vi "random_average_activity_11.vi"() -> ()   [LabVIEW 2025]
panel:
  in  "Enable":bool
  out "RandomSignal":dbl(graph)
  # "off"
  # "on"
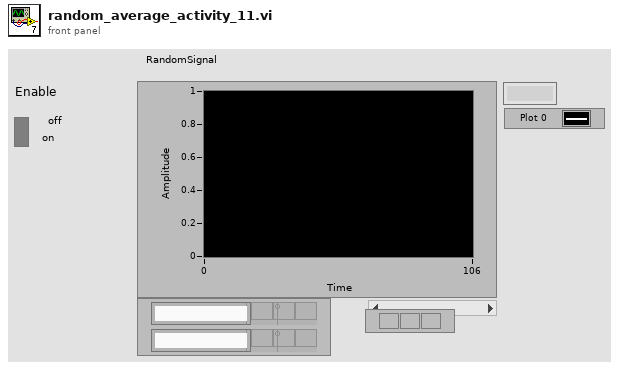
[diagram p1: front panel]
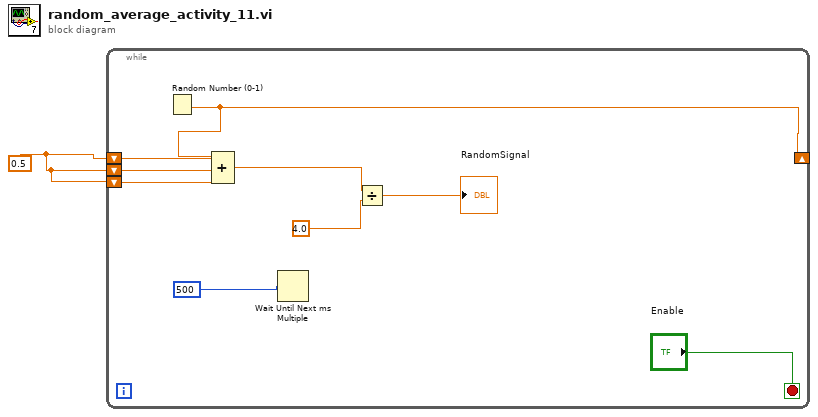
[diagram p0: block diagram]
diagram:
  w1 = 0.5
  n1 = while {
    shift-right: [w2] -> _
    shift-left: w1 -> [w3]
    shift-left: w1 -> [w4]
    shift-left: w1 -> [w5]
    stop <- "Enable" stop-if-true
    n2 = Random Number (0-1)() -> (number: 0 to 1=w2:dbl)
    n3 = Compound Arithmetic op=ADD(w2, w3, w4, w5) -> (w6:dbl)
    n4 = Wait Until Next ms Multiple(millisecond multiple=500) -> ()  [unwired: 1 out]
    n5 = Divide(x=w6, y=4.0) -> (x/y=→"RandomSignal":dbl)
  }
